vi "SplineHelp_GetQuinticSplinesFromWayPts.vi"(11 "WayPoints":T1[](array[typedef]) {"ROTATION"."SIN" format="%13.4f"; "ROTATION"."COS" format="%13.4f"; "ROTATION"."VALUE" format="%13.4f"; "TRANSLATION"."Y" format="%14.3f"; "TRANSLATION"."X" format="%14.3f"}) -> (0 "out Error":errorcluster, 3 "Splines":T4[](array[typedef]))   [LabVIEW 2019, in "Trajectory_Library.lvlib"]
doc: "Returns quintic splines from a set of waypoints.\n\nParameters:\n - waypoints - The array of waypoints (Translation)\n\nReturns:\n - Splines - Array of splines"
uses:
  Trajectory_Library.lvlib
  TypeDef/SPLINE.ctl
  <vilib>/Analysis/Matrix/Datatypes/RealMatrix.ctl
  TypeDef/POSE2D.ctl
  TypeDef/TRANSLATION2D.ctl
  TypeDef/ROTATION2D.ctl
  Util_CalcDist.vi
  <vilib>/Analysis/Matrix/NI_Matrix.lvlib
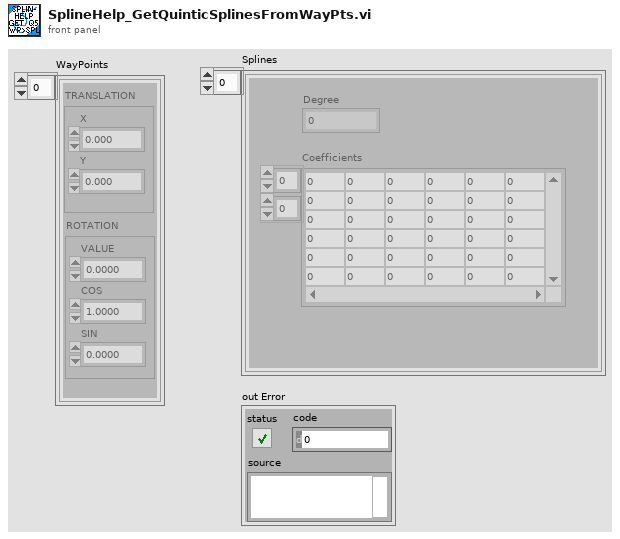
[diagram p1: front panel]
types:
  T1 = typedef "Trajectory_Library.lvlib/POSE2D.ctl" = cluster{"TRANSLATION":T2, "ROTATION":T3}
  T2 = typedef "Trajectory_Library.lvlib/TRANSLATION2D.ctl" = cluster{"X":dbl, "Y":dbl}
  T3 = typedef "Trajectory_Library.lvlib/ROTATION2D.ctl" = cluster{"VALUE":dbl, "COS":dbl, "SIN":dbl}
  T4 = typedef "Trajectory_Library.lvlib/SPLINE.ctl" = cluster{"Degree":i32, "Coefficients":T5}
  T5 = typedef "NI_Matrix.lvlib/RealMatrix.ctl" = dbl[][]
  T6 = typedef "Trajectory_Library.lvlib/SPLINE_CTRL_VECTOR.ctl" = cluster{"Xs":dbl[], "Ys":dbl[]}
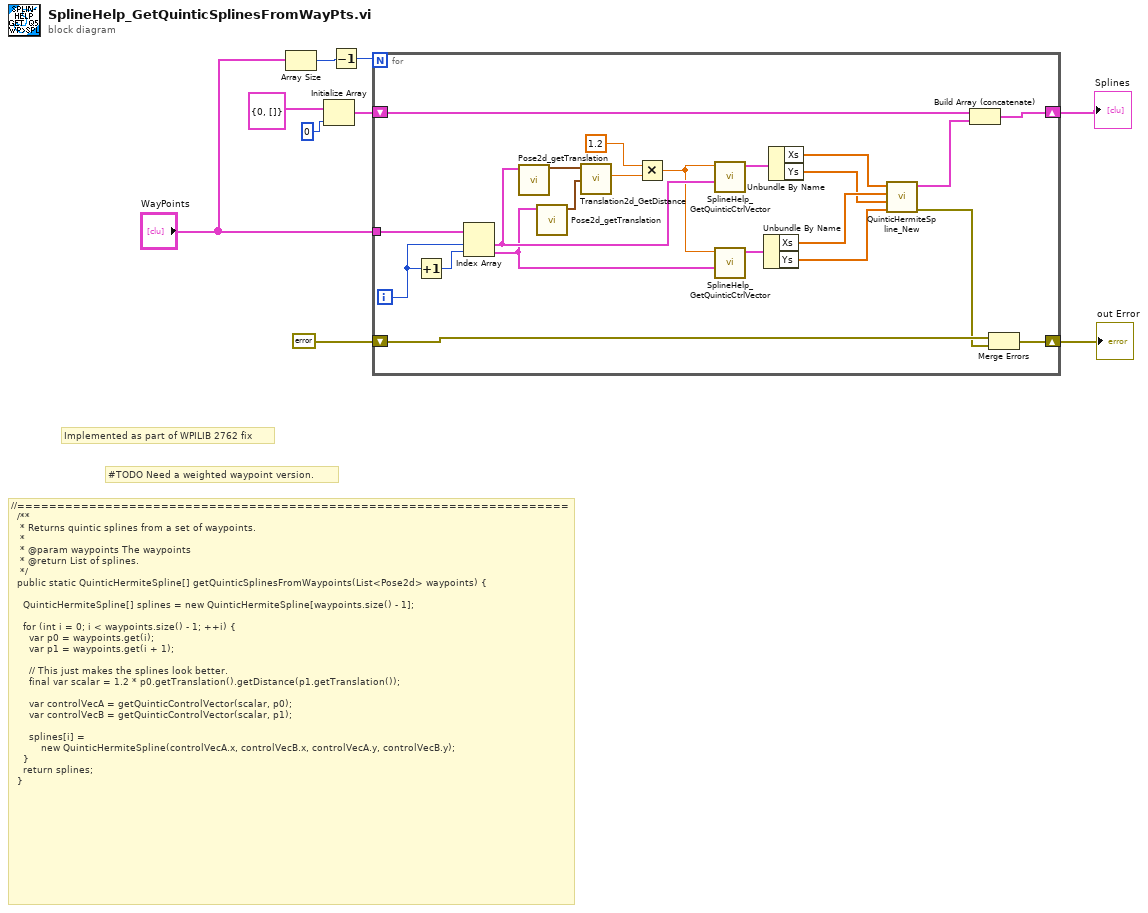
[diagram p0: block diagram]
diagram:
  # "#TODO Need a weighted waypoint version."
  # "//=====================================================================\n  /**\n   * Returns quintic splines from a set of waypoints.\n   *\n   * @param waypoints The waypoints\n   * @return List of splines.\n   */\n  public static QuinticHermiteSpline[] getQuinticSplinesFromWaypoints(List<Pose2d> waypoints) {\n\n    QuinticHermiteSpline[] splines = new QuinticHermiteSpline[waypoints.size() - 1];\n\n    for (int i = 0; i < waypoints.size() - 1; ++i) {\n      var p0 = waypoints.get(i);\n      var p1 = waypoints.get(i + 1);\n\n      // This just makes the splines look better.\n      final var scalar = 1.2 * p0.getTranslation().getDistance(p1.getTranslation());\n\n      var controlVecA = getQuinticControlVector(scalar, p0);\n      var controlVecB = getQuinticControlVector(scalar, p1);\n\n      splines[i] =\n          new QuinticHermiteSpline(controlVecA.x, controlVecB.x, controlVecA.y, controlVecB.y);\n    }\n    return splines;\n  }"
  # "Implemented as part of WPILIB 2762 fix"
  n1 = Array Size(array="WayPoints") -> (size(s)=w8:i32)
  n2 = Initialize Array(T4 {"Degree"=0, "Coefficients"=[]} ("SPLINE"), 0 ("dimension size")) -> (w5:T4[])
  n3 = Decrement(x=w8) -> (x-1=w9:i32)
  n4 = for {
    N: w9 -> [_]
    tunnel: "WayPoints" -> [w29]
    shift-right: [w20] -> w3
    shift-left: w5 -> [w24]
    shift-right: [w18] -> w1
    shift-left: errorcluster {"status"=FALSE, "code"=0, "source"=""} ("error constant") -> [w17]
    i -> [w21]
    n5 = Increment(x=w21) -> (x+1=w30:i32)
    n6 = Index Array(array=w29, index #1=w21, index #2=w30) -> (element #1=w26:T1, element #2=w22:T1)
    n7 = call "Pose2d_getTranslation.vi"("in POSE"=w26) -> ("outTRANSLATION"=w27:T2)  [unwired: 10 in]
    n8 = call "Pose2d_getTranslation.vi"("in POSE"=w22) -> ("outTRANSLATION"=w25:T2)  [unwired: 10 in]
    n9 = call "Translation2d_GetDistance.vi"("other Translation"=w25, "In Translation"=w27) -> ("Distance"=w28:dbl)  [unwired: 9 in]
    n10 = Multiply(x=1.2, y=w28) -> (x*y=w23:dbl)
    n11 = call "SplineHelp_GetQuinticCtrlVector.vi"("Input POSE"=w26, "Scalar"=w23) -> ("resultSpline_Ctrl_Vector"=w14:T6)  [unwired: 9 in]
    n12 = call "SplineHelp_GetQuinticCtrlVector.vi"("Input POSE"=w22, "Scalar"=w23) -> ("resultSpline_Ctrl_Vector"=w15:T6)  [unwired: 9 in]
    n13 = Unbundle By Name(w15) -> ("Xs"=w12:dbl[], "Ys"=w10:dbl[])
    n14 = Unbundle By Name(w14) -> ("Xs"=w13:dbl[], "Ys"=w11:dbl[])
    n15 = call "QuinticHermiteSpline_New.vi"("yFinalCtrlVector"=w10, "yInitialCtrlVector"=w11, "xFinalCtrlVector"=w12, "XInitialCtrlVector"=w13) -> ("error out"=w16:errorcluster, "QuinticHermiteSpline"=w19:T4)  [unwired: 6 in]
    n16 = Build Array (concatenate)(w24, w19) -> (w20:T4[])
    n17 = Merge Errors(w17, w16) -> (w18:errorcluster)
  }
  "Splines" <- w3
  "out Error" <- w1
